vi "P_REG.vi"(0 "milliseconds to wait":u32, 1 "Coerce?":bool, 2 "History Data in":dbl[](array[numeric]), 5 "element":T4, 7 "Default værdier":T2, 9 "SP":dbl, 12 "History Data 2":dbl[](array[numeric]), 13 "Tout":dbl, 14 "P?":bool) -> (4 "Cluster":T3, 6 "History Data":dbl[](array[numeric]), 8 "Tout out":dbl, 15 "P I D":T1)   [LabVIEW 2022 SP3]
uses:
  TypeDefs/P_I_D_Data_type.ctl
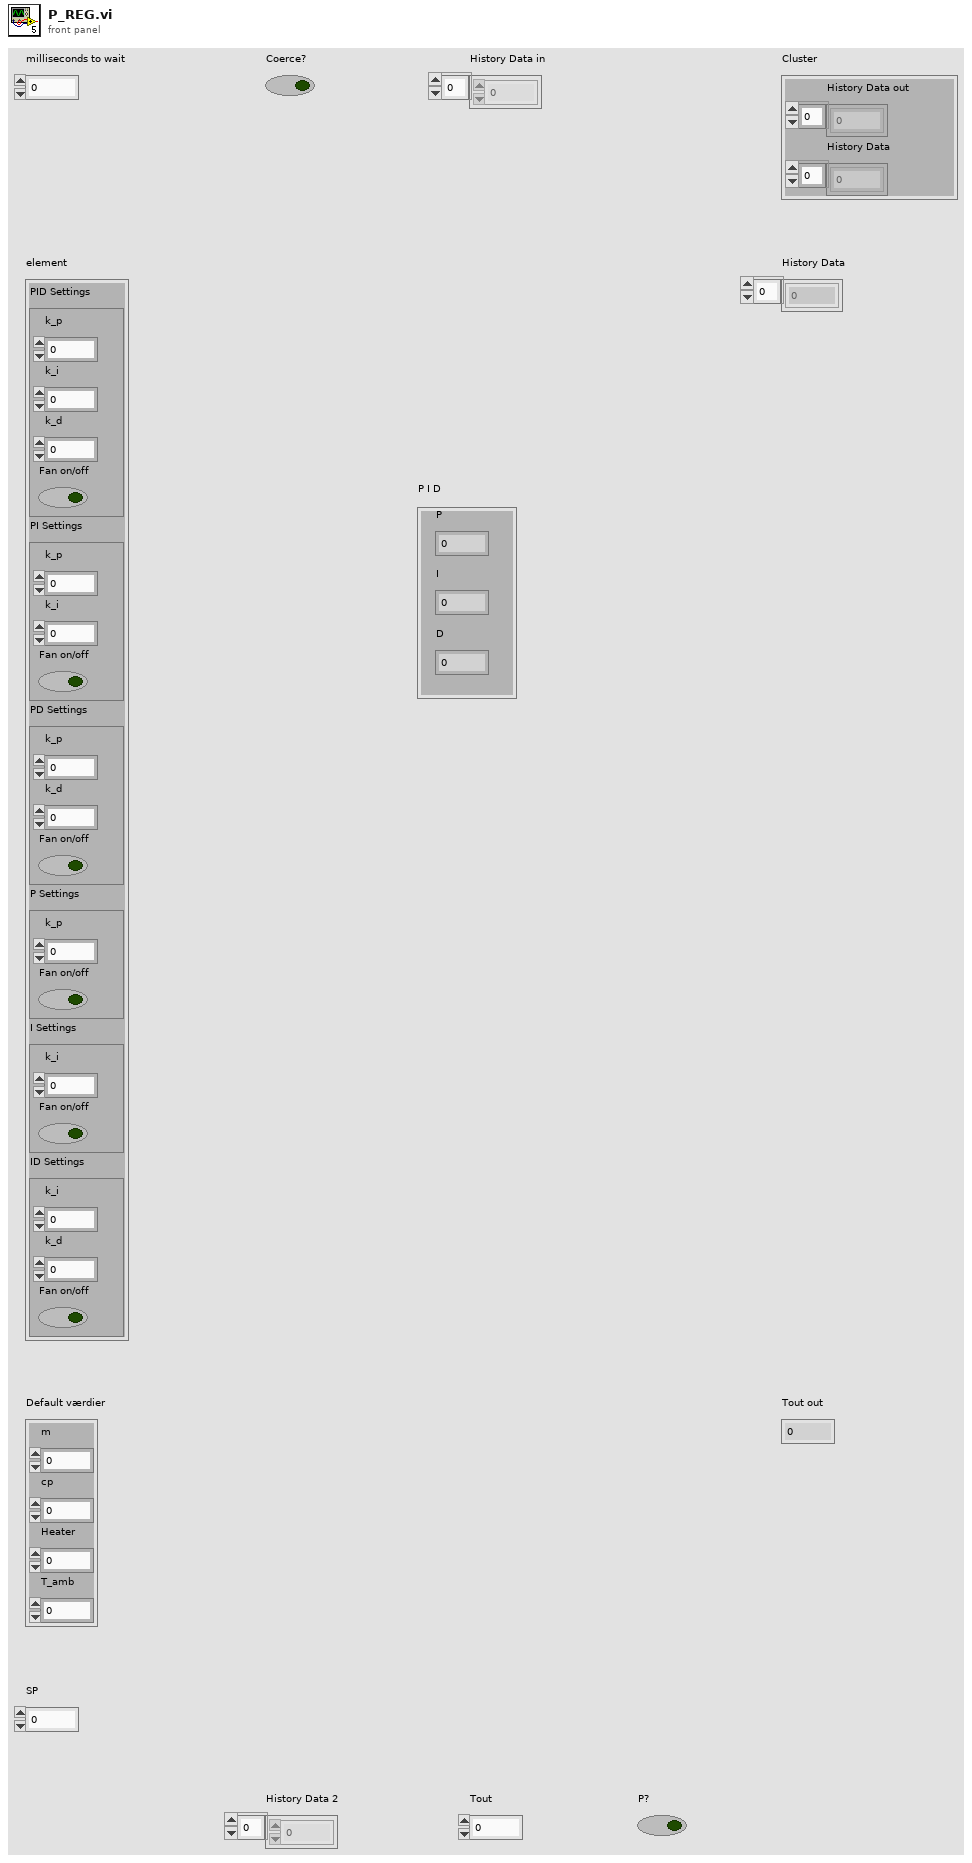
[diagram p1: front panel]
types:
  T1 = typedef "P_I_D_Data_type.ctl" = cluster{"P":dbl, "I":dbl, "D":dbl}
  T2 = cluster{"m":dbl, "cp":dbl, "Heater":dbl, "T_amb":dbl}
  T3 = cluster{"History Data out":dbl[], "History Data":dbl[]}
  T4 = cluster{"PID Settings":cluster{"k_p":dbl, "k_i":dbl, "k_d":dbl, "Fan on/off":bool}, "PI Settings":cluster{"k_p":dbl, "k_i":dbl, "Fan on/off":bool}, "PD Settings":cluster{"k_p":dbl, "k_d":dbl, "Fan on/off":bool}, "P Settings":cluster{"k_p":dbl, "Fan on/off":bool}, "I Settings":cluster{"k_i":dbl, "Fan on/off":bool}, "ID Settings":cluster{"k_i":dbl, "k_d":dbl, "Fan on/off":bool}}
  T5 = enum16{"I_REG", "ID_REG", "P_REG", "PI_REG", "PD_REG", "PID_REG"}
  T6 = cluster{"History Data in":dbl[], "History Data 2":dbl[]}
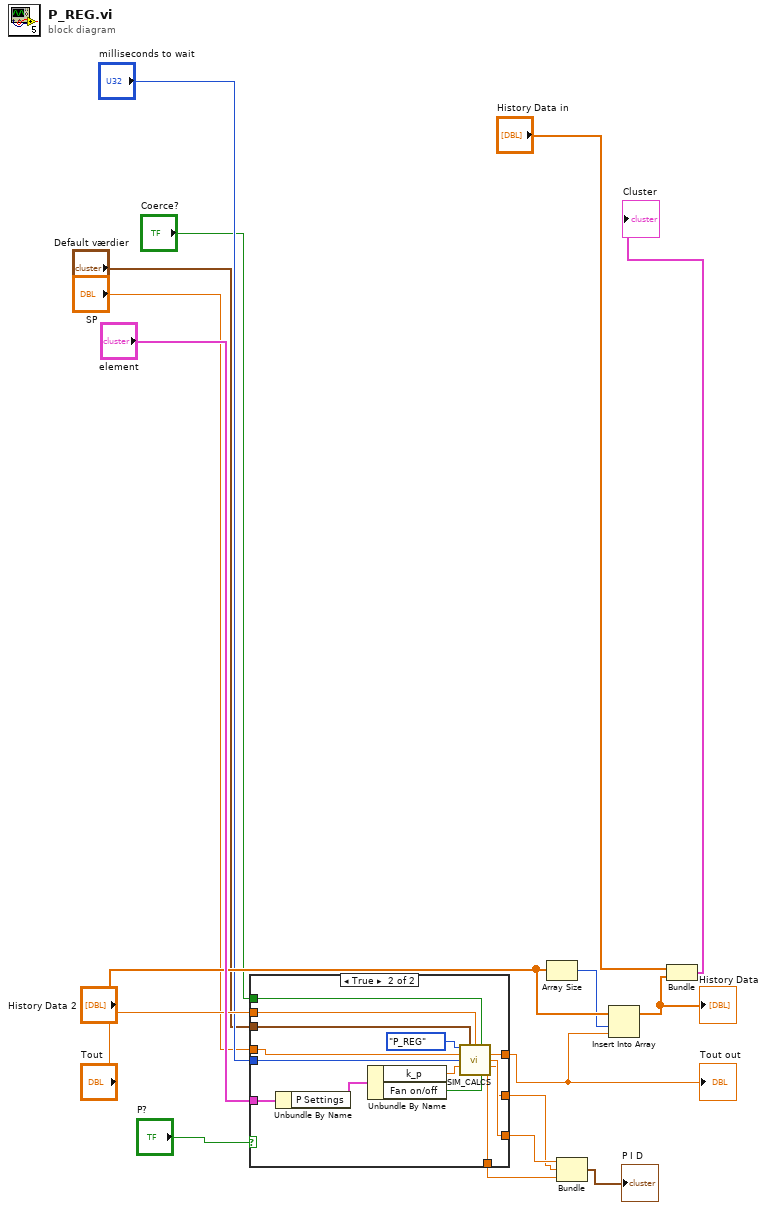
[diagram p0: block diagram]
diagram:
  n1 = case shown="True" "P?" {
    tunnel: "Tout" -> [_ w30]
    tunnel: "Default værdier" -> [_ w29]
    tunnel: [_ w27] -> w11
    tunnel: "milliseconds to wait" -> [_ w24]
    tunnel: "Coerce?" -> [_ w23]
    tunnel: "SP" -> [_ w22]
    tunnel: "element" -> [_ w21]
    tunnel: [_ w20] -> w4
    tunnel: [_ w19] -> w3
    tunnel: [_ w18] -> w2
    frame False {
    }
    frame True {
      n2 = Unbundle By Name(w21) -> ("P Settings"=w26:cluster{"k_p":dbl, "Fan on/off":bool})
      n3 = Unbundle By Name(w26) -> ("k_p"=w31:dbl, "Fan on/off"=w28:bool)
      n4 = call "SIM_CALCS.vi"("Regulation type"=T5."P_REG", "Default værdier"=w29, "Tout in"=w30, "Coerce?"=w23, "SP"=w22, "milliseconds to wait"=w24, "k_p"=w31, "Fan on/off"=w28) -> ("Tout out"=w27:dbl, "P"=w20:dbl, "I"=w19:dbl, "D"=w18:dbl)  [unwired: 3 in, 1 out]
    }
  }
  "Tout out" <- w11
  n5 = Array Size(array="History Data 2") -> (size(s)=w10:i32)
  n6 = Bundle("P"=w4, "I"=w3, "D"=w2) -> (→"P I D":cluster{"P":dbl, "I":dbl, "D":dbl})  [unwired: 1 in]
  n7 = Insert Into Array(array="History Data 2", index=w10, new element=w11) -> (w13:dbl[])
  "History Data" <- w13
  n8 = Bundle("History Data in"="History Data in", "History Data 2"=w13) -> (→"Cluster":T6)  [unwired: 1 in]
